vi "Apex view loop error handler.vi"(8 "errors in":errorcluster[](array[cluster])) -> (0 "error out":errorcluster)   [LabVIEW 2018]
doc: "This VI handles all errors in the View loop. Since some event cases might loop many times, with loops that want to run even if other loops have errors, it has an array input. \n\nIts main feature is that if an error occurs (and isn't ignored) on a regular basis (default = 3 times in 5 seconds), then a delay (default 2 seconds) is added to allow the user time to attempt to deal with the source of the errors without being bombarded with popups."
uses:
  <userlib>/nLight Error Handling/Merge errors no loss.vi
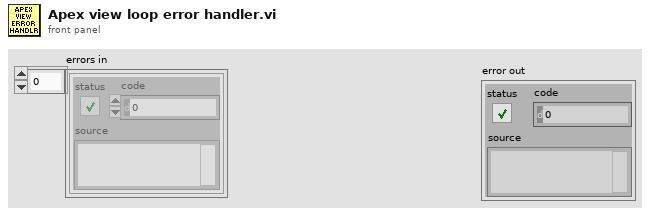
[diagram p1: front panel]
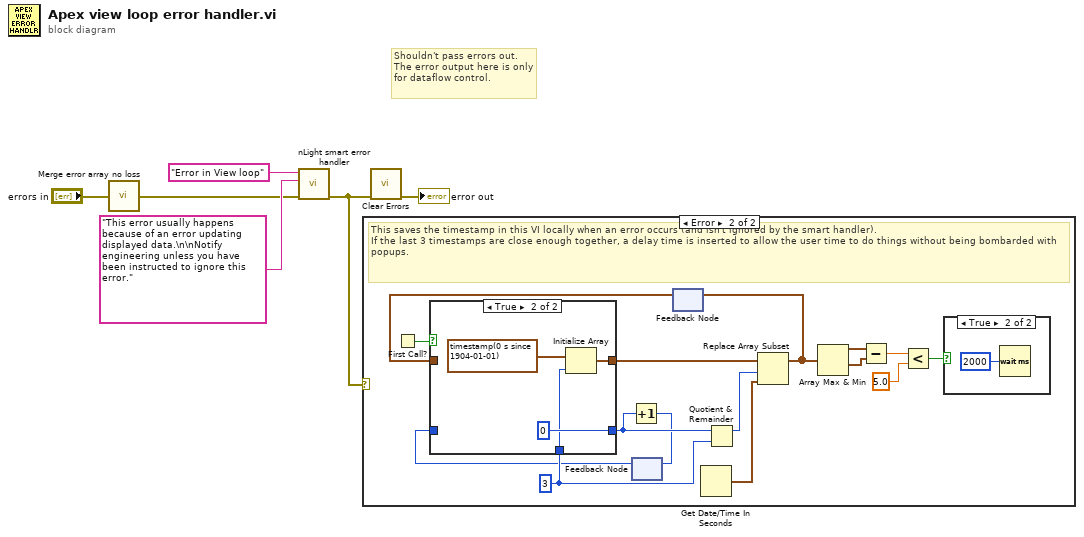
[diagram p0: block diagram]
diagram:
  # "Shouldn't pass errors out.  The error output here is only for dataflow control."
  n1 = call <userlib>:"Merge error array no loss.vi"("error array in"="errors in") -> ("error out"=w2:errorcluster)
  n2 = call <userlib>:"nLight smart error handler.vi"("error in (no error)"=w2, "Popup message if not in table (Generic message)"="This error usually happens because of an error updating displayed data.\n\nNotify engineering unless you have been instructed to ignore this error.", "Error title if not in table [<40 chars] (\"LabVIEW error\")"="Error in View loop" ("Error title if not in table [<40 chars] (\"LabVIEW error\")")) -> ("error out"=w3:errorcluster)  [unwired: 6 in, 2 out]
  n3 = case shown="Error" w3 {
    frame No Error {
    }
    frame Error {
      w18 = 3 ("dimension size")
      # "This saves the timestamp in this VI locally when an error occurs (and isn't ignored by the smart handler).\nIf the last 3 timestamps are close enough together, a delay time is inserted to allow the user time to do things without being bombarded with popups."
      n4 = First Call?() -> (First Call?: T/F=w19:bool)
      n5 = feedback #1() -> (w13:i32)  [unwired: 1 in]
      n6 = feedback #2() -> (w16:timestamp[])  [unwired: 1 in]
      n7 = case shown="True" w19 {
        tunnel: [w24 w27] -> w21
        tunnel: [w23 0] -> w15
        tunnel: w18 -> [_ w25]
        tunnel: w16 -> [w24 _]
        tunnel: w13 -> [w23 _]
        frame False {
        }
        frame True {
          n8 = Initialize Array(timestamp(0 s since 1904-01-01) ("current time"), w25) -> (w27:timestamp[])
        }
      }
      n9 = Increment(x=w15) -> (x+1=w14:i32)
      n10 = feedback-in #1(w14) -> ()
      n11 = Get Date/Time In Seconds() -> (seconds since 1Jan1904=w20:timestamp)
      n12 = Quotient & Remainder(x=w15, y=w18) -> (x-y*floor(x/y)=w17:i32)  [unwired: 1 out]
      n13 = Replace Array Subset(array=w21, new element=w20, index=w17) -> (w12:timestamp[])
      n14 = feedback-in #2(w12) -> ()
      n15 = Array Max & Min(array=w12) -> (max value=w11:timestamp, min value=w10:timestamp)  [unwired: 2 out]
      n16 = Subtract(x=w11, y=w10) -> (x-y=w9:dbl)
      n17 = Less?(x=w9, y=5.0) -> (x < y?=w7:bool)
      n18 = case shown="True" w7 {
        frame False {
        }
        frame True {
          n19 = Wait (ms)(milliseconds to wait=u32 2000) -> ()  [unwired: 1 out]
        }
      }
    }
  }
  n20 = call <vilib>:"Clear Errors.vi"("error in (no error)"=w3) -> ("error out"=→"error out":errorcluster)  [unwired: 5 in, 1 out]
